vi "Add APU Angle RTM.vi"(8 "error in (no error)":errorcluster, 11 "Node Ptr":u64 format="%.0x") -> (0 "error out":errorcluster)   [LabVIEW 2011, in "Engine Sim System Explorer.lvlib"]
uses:
  Engine Sim System Explorer.lvlib
  TypeDefs/APUComp.ctl
  <vilib>/NI Veristand/Custom Device API/Custom Device Channel.ctl
  <vilib>/NI Veristand/Custom Device API/Custom Device Channel Type.ctl
  Shared/Engine Simulation Global.vi
  <vilib>/NI Veristand/Custom Device API/Get Item Property (Variant).vi
  Engine Simulation Shared.lvlib
  <vilib>/NI Veristand/Custom Device API/Custom Device API.lvlib
  <vilib>/NI Veristand/Custom Device Tools/Custom Device Utility Library/Custom Device Utility Library.lvlib
panel:
  in  "Tag":string
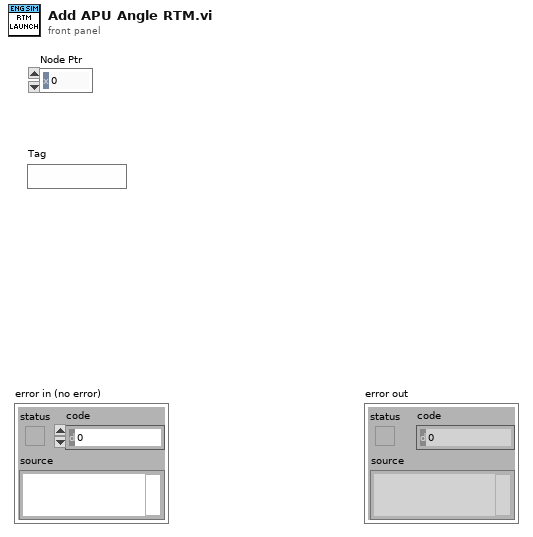
[diagram p1: front panel]
types:
  T1 = typedef "Custom Device API.lvlib/Custom Device Channel.ctl" = cluster{"Type":T2, "Units":string, "Default Value":dbl, "Faultable":bool, "Scalable":bool}
  T2 = typedef "Custom Device API.lvlib/Custom Device Channel Type.ctl" = enum16{"Input", "Output"}
  T3 = typedef "Engine Sim System Explorer.lvlib/APUComp.ctl" = cluster{"Crank Angle":bool, "Cycle Angle":bool, "Reset":bool}
  T4 = typedef "Custom Device API.lvlib/Custom Device Item Ref.ctl" = u64
  T5 = typedef "Custom Device API.lvlib/Custom Device Item Info.ctl" = cluster{"Name":string, "Is Channel":bool, "GUID":string}
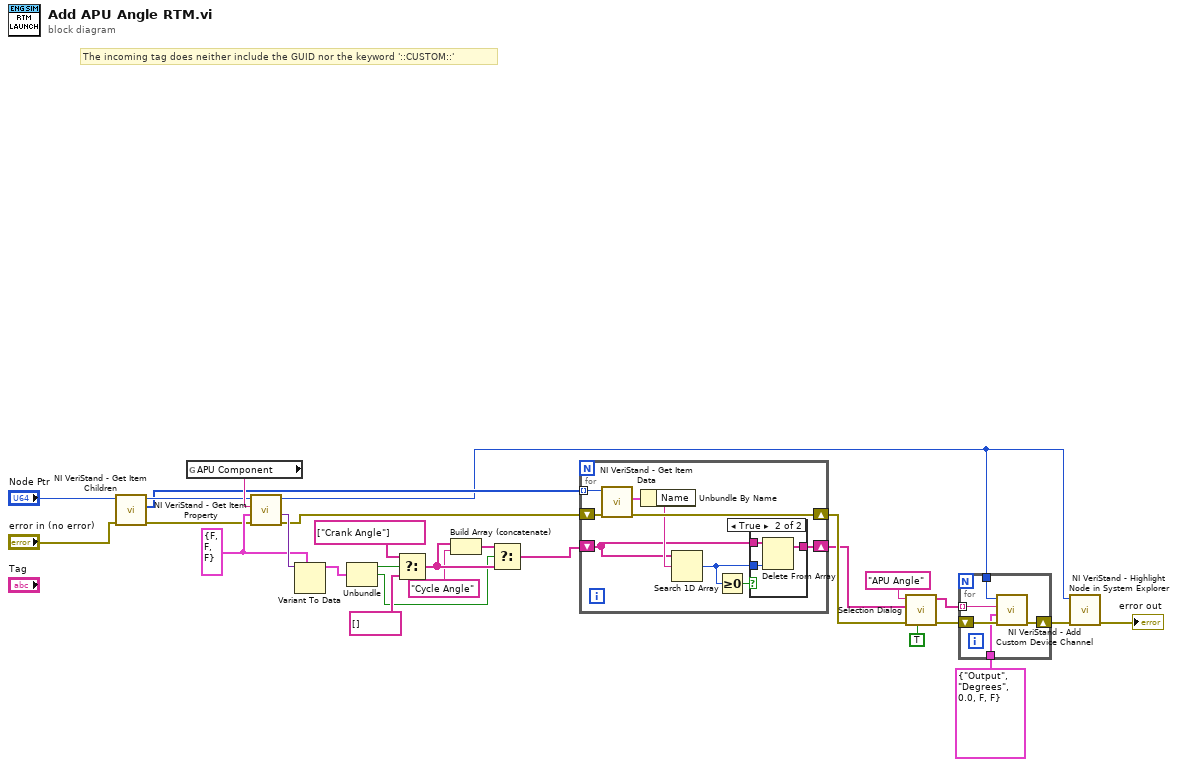
[diagram p0: block diagram]
diagram:
  w26 = T3 {"Crank Angle"=FALSE, "Cycle Angle"=FALSE, "Reset"=FALSE}
  # "The incoming tag does neither include the GUID nor the keyword '::CUSTOM::'"
  n1 = call <vilib>:"NI VeriStand - Get Item Children.vi"("error in (no error)"="error in (no error)", "Item Ref in"="Node Ptr") -> ("error out"=w23:errorcluster, "Child Refs"=w24:T4[], "Item Ref out"=w25:T4)  [unwired: 6 in, 1 out]
  n2 = global read "Engine Simulation Global.vi" "APU Component"() -> (w28:string)
  n3 = call-poly <vilib>:"NI VeriStand - Get Item Property.vi"("error in (no error)"=w23, "Default Value"=w26, "Property Name"=w28, "Item Ref in"=w25) -> ("error out"=w3:errorcluster, "Value"=w27:variant, "Item Ref out"=w4:T4)  [unwired: 4 in, 1 out]
  n4 = Variant To Data(type=w26, Variant=w27) -> (data=w12:T3)  [unwired: 1 in, 1 out]
  n5 = Unbundle(w12) -> ("Crank Angle"=w11:bool, "Cycle Angle"=w7:bool)  [unwired: 1 out]
  n6 = Select(t=string[] ["Crank Angle"], s=w11, f=string[] []) -> (s? t:f=w8:string[])
  n7 = Build Array (concatenate)(w8, "Cycle Angle" ("Name")) -> (w5:string[])
  n8 = Select(t=w5, s=w7, f=w8) -> (s? t:f=w2:string[])
  n9 = for {
    tunnel: w24 -> [w37] mode=indexing
    shift-right: [w35] -> w20
    shift-left: w3 -> [w34]
    shift-right: [w32] -> w1
    shift-left: w2 -> [w30]
    n10 = call <vilib>:"NI VeriStand - Get Item Data.vi"("error in (no error)"=w34, "Item Ref in"=w37) -> ("error out"=w35:errorcluster, "Item Info"=w36:T5)  [unwired: 6 in, 2 out]
    n11 = Unbundle By Name(w36) -> ("Name"=w31:string)
    n12 = Search 1D Array(1D array=w30, element=w31) -> (index of element=w29:i32)  [unwired: 1 in]
    n13 = Greater Or Equal To 0?(x=w29) -> (x >= 0?=w33:bool)
    n14 = case shown="True" w33 {
      tunnel: [w38 w40] -> w32
      tunnel: w30 -> [w38 w41]
      tunnel: w29 -> [_ w39]
      frame False {
      }
      frame True {
        n15 = Delete From Array(array=w41, index=w39) -> (array with subset deleted=w40:string[])  [unwired: 1 in, 1 out]
      }
    }
  }
  n16 = call "Selection Dialog.vi"("Multi-Selection?"=TRUE, "error in (no error)"=w20, "Tree Items"=w1, "Root Tag"="APU Angle") -> ("error out"=w18:errorcluster, "Selected Names"=w19:string[])  [unwired: 5 in, 1 out]
  n17 = for {
    tunnel: w19 -> [w45] mode=indexing
    shift-right: [w42] -> w14
    shift-left: w18 -> [w46]
    tunnel: w4 -> [w44]
    tunnel: T1 {"Type"=enum."Output", "Units"="Degrees", "Default Value"=0.0, "Faultable"=FALSE, "Scalable"=FALSE} ("Channel") -> [w43]
    n18 = call <vilib>:"NI VeriStand - Add Custom Device Channel.vi"("error in (no error)"=w46, "Channel"=w43, "Channel Name"=w45, "Parent Ref in"=w44) -> ("error out"=w42:errorcluster)  [unwired: 4 in, 3 out]
  }
  n19 = call <vilib>:"NI VeriStand - Highlight Node in System Explorer.vi"("error in (no error)"=w14, "Item Ref in"=w4) -> ("error out"=→"error out":errorcluster)  [unwired: 8 in, 1 out]
